vi "M method_avg (SubVI).vi"(5 "Tc (mSec)":u32 format="%#_6f", 7 "Tick Count (mSec)":u32 format="%#_6f", 8 "Encoder velocity_pre (pulse/s)":fxp<+/-,32,16>, 9 "Shift Register in 2":i32 format="%#_6f", 10 "Shift Register in 1":u32 format="%#_6f", 11 "Encoder pulses":i32 format="%#_6f") -> (0 "Encoder velocity (pulse/s)":fxp<+/-,32,16>, 1 "Shift Register out 2":i32 format="%#_6f", 2 "Shift Register out 1":u32 format="%#_6f")   [LabVIEW 2014]
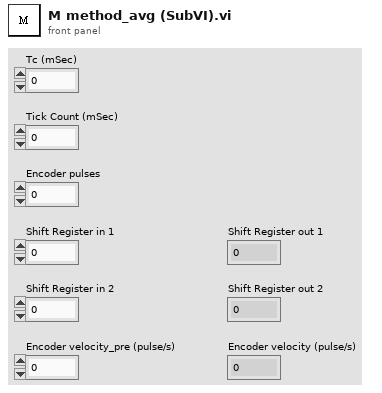
[diagram p1: front panel]
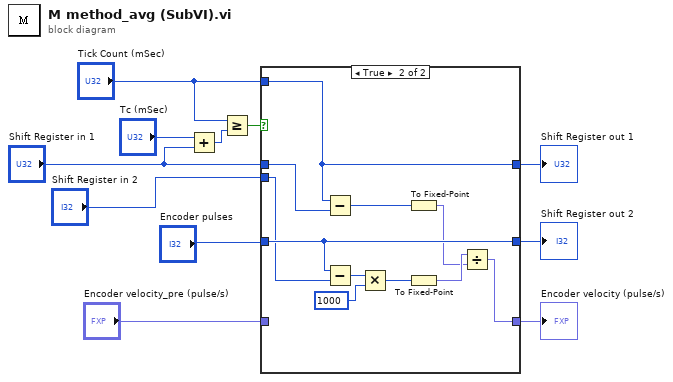
[diagram p0: block diagram]
diagram:
  n1 = Add(x="Tc (mSec)", y="Shift Register in 1") -> (x+y=w4:u32)
  n2 = Greater Or Equal?(x="Tick Count (mSec)", y=w4) -> (x >= y?=w3:bool)
  n3 = case shown="True" w3 {
    tunnel: [w14 w25] -> w5
    tunnel: "Tick Count (mSec)" -> [_ w25]
    tunnel: "Shift Register in 1" -> [w14 w24]
    tunnel: [w13 w23] -> w8
    tunnel: "Encoder pulses" -> [_ w23]
    tunnel: "Shift Register in 2" -> [w13 w22]
    tunnel: [w12 w15] -> w2
    tunnel: "Encoder velocity_pre (pulse/s)" -> [w12 _]
    frame False {
    }
    frame True {
      n4 = Subtract(x=w25, y=w24) -> (x-y=w19:u32)
      n5 = Subtract(x=w23, y=w22) -> (x-y=w21:i32)
      n6 = Multiply(x=w21, y=1000) -> (x*y=w18:i32)
      n7 = To Fixed-Point(number=w19) -> (fixed-point=w16:fxp<+,32,32>)  [unwired: 1 in]
      n8 = To Fixed-Point(number=w18) -> (fixed-point=w17:fxp<+/-,32,32>)  [unwired: 1 in]
      n9 = Divide(x=w17, y=w16) -> (x/y=w15:fxp<+/-,32,16>)
    }
  }
  "Shift Register out 2" <- w8
  "Shift Register out 1" <- w5
  "Encoder velocity (pulse/s)" <- w2
